vi "Sample Channel.vi"(8 "error in (no error)":errorcluster, 11 "Node Ptr":T1 format="%.0x") -> (0 "error out":errorcluster)   [LabVIEW 2015, in "Import Export Sample Custom Device System Explorer.lvlib"]
uses:
  Import Export Sample Custom Device System Explorer.lvlib
  <vilib>/NI Veristand/Custom Device API/Custom Device Item Ref.ctl
  <vilib>/NI Veristand/Custom Device API/Get Item Property (String).vi
  <vilib>/NI Veristand/Custom Device API/Set Item Property (String).vi
  <vilib>/NI Veristand/Custom Device API/Custom Device API.lvlib
panel:
  in  "Units":string
  in  "Header":cluster{"Section Name":string}={"Section Name"="Custom Device Item Settings"}
  in  "Description":string
  in  "Name":string
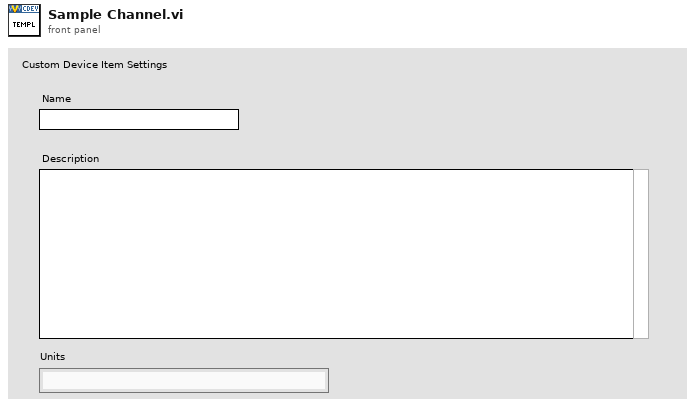
[diagram p1: front panel]
types:
  T1 = typedef "Custom Device API.lvlib/Custom Device Item Ref.ctl" = u64
  T2 = typedef "Custom Device API.lvlib/Custom Device Item Info.ctl" = cluster{"Name":string, "Is Channel":bool, "GUID":string, "Is Waveform":bool}
  T3 = typedef "Custom Device API.lvlib/Custom Device Commands.ctl" = enum16{"Default", "Item renamed", "Shutdown", "Dynamic button pressed"}
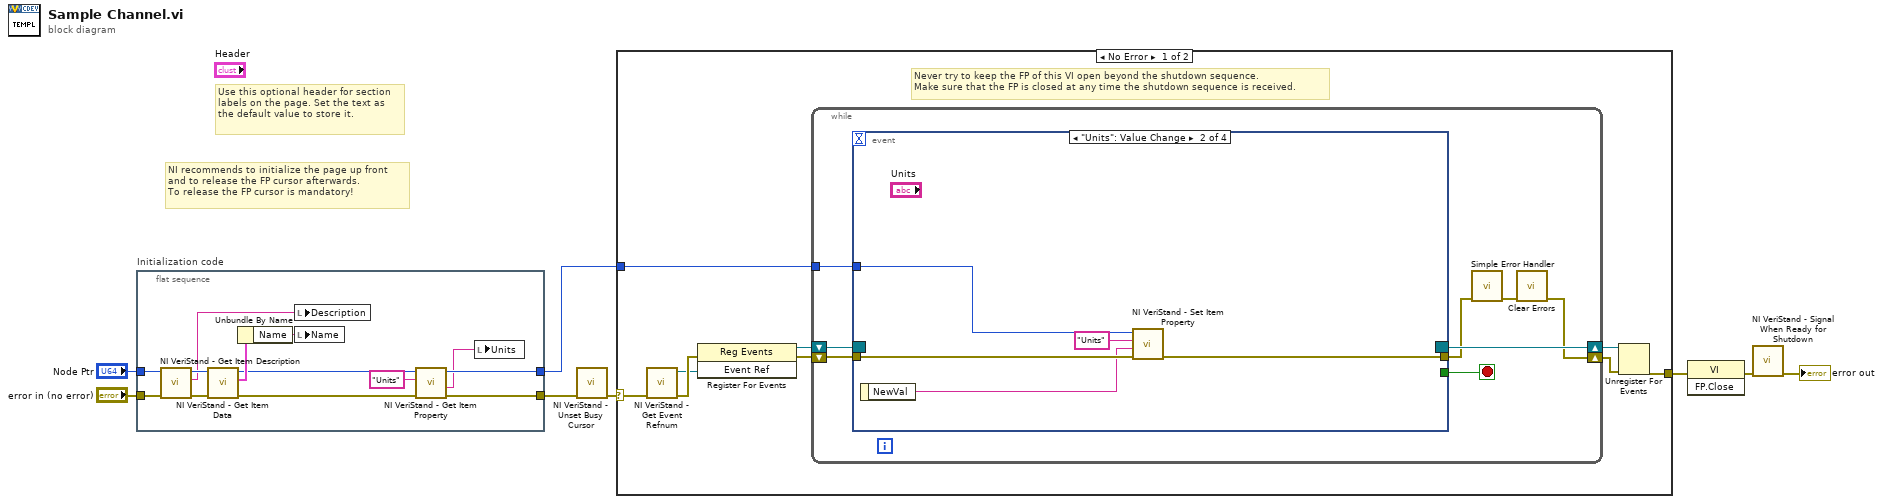
[diagram p0: block diagram]
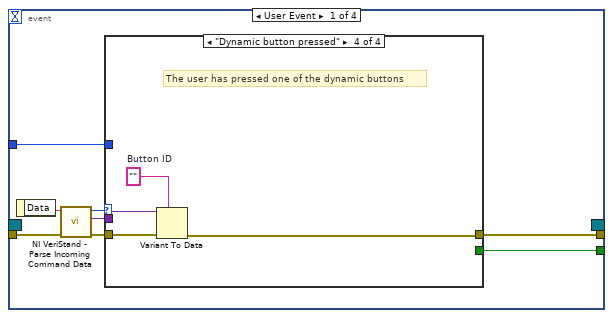
[diagram p2: hidden frame]
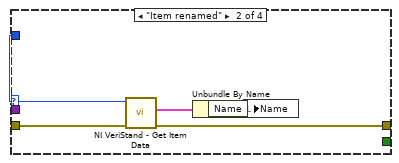
[diagram p4: hidden frame]
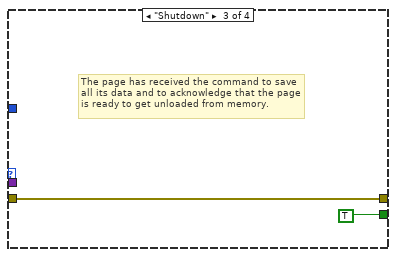
[diagram p5: hidden frame]
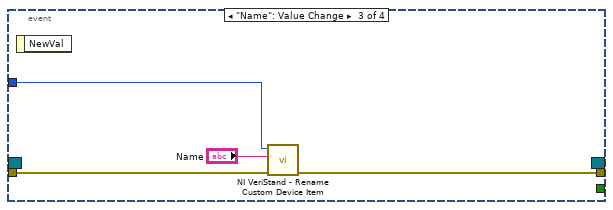
[diagram p6: hidden frame]
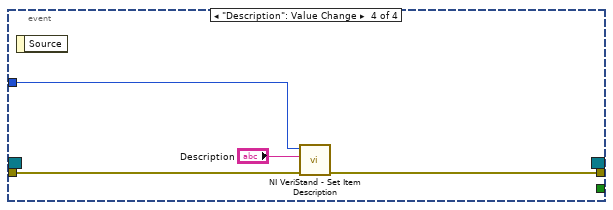
[diagram p7: hidden frame]
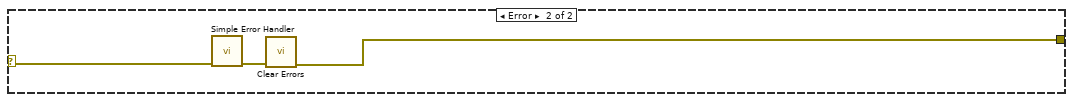
[diagram p8: hidden frame]
diagram:
  # "Use this optional header for section labels on the page. Set the text as the default value to store it."
  # "NI recommends to initialize the page up front\nand to release the FP cursor afterwards.\nTo release the FP cursor is mandatory!"
  n1 = flat-sequence "Initialization code" {
    tunnel: "error in (no error)" -> [w20]
    tunnel: "Node Ptr" -> [w19]
    tunnel: [w12] -> w4
    tunnel: [w11] -> w1
    frame #0 {
      n2 = call <vilib>:"NI VeriStand - Get Item Description.vi"("error in (no error)"=w20, "Item Ref in"=w19) -> ("error out"=w17:errorcluster, "Description"=w18:string, "Item Ref out"=w21:T1)  [unwired: 7 out]
      n3 = call <vilib>:"NI VeriStand - Get Item Data.vi"("error in (no error)"=w17, "Item Ref in"=w21) -> ("error out"=w13:errorcluster, "Item Info"=w16:T2, "Item Ref out"=w14:T1)  [unwired: 7 out]
      n4 = Unbundle By Name(w16) -> ("Name"=w15:string)
      n5 = local write "Description"(w18) -> ()
      n6 = local write "Name"(w15) -> ()
      n7 = call-poly <vilib>:"NI VeriStand - Get Item Property.vi"("error in (no error)"=w13, "Property Name"="Units", "Item Ref in"=w14) -> ("error out"=w12:errorcluster, "Value"=w10:string, "Item Ref out"=w11:T1)  [unwired: 5 in, 1 out]
      n8 = local write "Units"(w10) -> ()
    }
  }
  n9 = call <vilib>:"NI VeriStand - Unset Busy Cursor.vi"("error in (no error)"=w4) -> ("error out"=w3:errorcluster)  [unwired: 10 out]
  n10 = case shown="No Error" w3 {
    selector: w3 -> [w22 w74]
    tunnel: [w27 w72] -> w8
    tunnel: w1 -> [w23 _]
    frame No Error {
      # "Never try to keep the FP of this VI open beyond the shutdown sequence.\nMake sure that the FP is closed at any time the shutdown sequence is received."
      n11 = call <vilib>:"NI VeriStand - Get Event Refnum.vi"("error in (no error)"=w22) -> ("error out"=w30:errorcluster, "Event Ref"=w26:refnum<user-event>)  [unwired: 9 out]
      n12 = register-events(error in=w30, w26) -> (reference out=w24:refnum<event-registration>, error out=w25:errorcluster)  [unwired: 1 in]
      n13 = while {
        tunnel: w23 -> [w34]
        shift-right: [w31] -> w28
        shift-left: w25 -> [w37]
        shift-right: [w38] -> w29
        shift-left: w24 -> [w36]
        stop <- w35 stop-if-true
        n14 = event shown="[1] \"Units\": Value Change" {
          selector: w36 -> [_ _ _ _]
          dyn-events: [_ _ _ _] -> w38
          timeout: _ -> [_ _ _ _]
          tunnel: w37 -> [w46 w62 w67 w70]
          tunnel: [w42 _ _ _] -> w35
          tunnel: [w41 w61 w66 w69] -> w33
          tunnel: w34 -> [w40 w63 w65 w71]
          event User Event {
            n15 = event-data() -> ("Data"=w45:string)  [unwired: 1 out]
            n16 = call <vilib>:"NI VeriStand - Parse Incoming Command Data.vi"("error in (no error)"=w46, "Incoming data"=w45) -> ("error out"=w44:errorcluster, "Outgoing data"=w39:variant, "Action"=w43:T3)  [unwired: 7 out]
            n17 = case shown="\"Dynamic button pressed\"" w43 {
              tunnel: w44 -> [w47 w52 w53 w58]
              tunnel: [_ _ TRUE _] -> w42
              tunnel: [w47 w49 w53 w55] -> w41
              tunnel: w40 -> [_ w51 _ _]
              tunnel: w39 -> [_ _ _ w57]
              frame "Default", Default {
              }
              frame "Item renamed" {
                n18 = call <vilib>:"NI VeriStand - Get Item Data.vi"("error in (no error)"=w52, "Item Ref in"=w51) -> ("error out"=w49:errorcluster, "Item Info"=w50:T2)  [unwired: 8 out]
                n19 = Unbundle By Name(w50) -> ("Name"=w48:string)
                n20 = local write "Name"(w48) -> ()
              }
              frame "Shutdown" {
                # "The page has received the command to save all its data and to acknowledge that the page is ready to get unloaded from memory."
              }
              frame "Dynamic button pressed" {
                w56 = ""  # Button ID
                # "The user has pressed one of the dynamic buttons"
                n21 = Variant To Data(error in=w58, type=w56, Variant=w57) -> (error out=w55:errorcluster)  [unwired: 1 out]
              }
            }
          }
          event "Units": Value Change {
            n22 = event-data() -> ("NewVal"=w59:string)  [unwired: 1 out]
            n23 = call-poly <vilib>:"NI VeriStand - Set Item Property.vi"("error in (no error)"=w62, "Value"=w59, "Property Name"="Units", "Item Ref in"=w63) -> ("error out"=w61:errorcluster)  [unwired: 5 in, 2 out]
          }
          event "Name": Value Change {
            n24 = event-data() -> ()  [unwired: 2 out]
            n25 = call <vilib>:"NI VeriStand - Rename Custom Device Item.vi"("error in (no error)"=w67, "New Name"="Name", "Item Ref in"=w65) -> ("error out"=w66:errorcluster)  [unwired: 1 in, 7 out]
          }
          event "Description": Value Change {
            n26 = event-data() -> ()  [unwired: 2 out]
            n27 = call <vilib>:"NI VeriStand - Set Item Description.vi"("error in (no error)"=w70, "Description"="Description", "Item Ref in"=w71) -> ("error out"=w69:errorcluster)  [unwired: 8 out]
          }
        }
        n28 = call <vilib>:"Simple Error Handler.vi"("error in (no error)"=w33) -> ("error out"=w32:errorcluster)  [unwired: 1 in, 7 out]
        n29 = call <vilib>:"Clear Errors.vi"("error in (no error)"=w32) -> ("error out"=w31:errorcluster)  [unwired: 1 in, 5 out]
      }
      n30 = Unregister For Events(event registration refnum=w29, error in=w28) -> (error out=w27:errorcluster)
    }
    frame Error {
      n31 = call <vilib>:"Simple Error Handler.vi"("error in (no error)"=w74) -> ("error out"=w73:errorcluster)  [unwired: 1 in, 7 out]
      n32 = call <vilib>:"Clear Errors.vi"("error in (no error)"=w73) -> ("error out"=w72:errorcluster)  [unwired: 1 in, 5 out]
    }
  }
  n33 = invoke class="VI" method="FP.Close"(error in=w8) -> (error out=w7:errorcluster)  [unwired: 2 in, 2 out]
  n34 = call <vilib>:"NI VeriStand - Signal When Ready for Shutdown.vi"("error in (no error)"=w7) -> ("error out"=→"error out":errorcluster)  [unwired: 10 out]
